vi "Annotate April.vi"(6 "hilight":bool, 7 "Annotate":bool, 9 "cutoffs":T1, 10 "Detected Tags":T3(array[cluster]), 11 "Refnum in":T2) -> (1 "margins":dbl[](array[numeric]), 2 "tags":T3(array[cluster]), 3 "Refnum out":T2)   [LabVIEW 2025]
uses:
  <vilib>/vision/Image Controls.llb/IMAQ Image.ctl
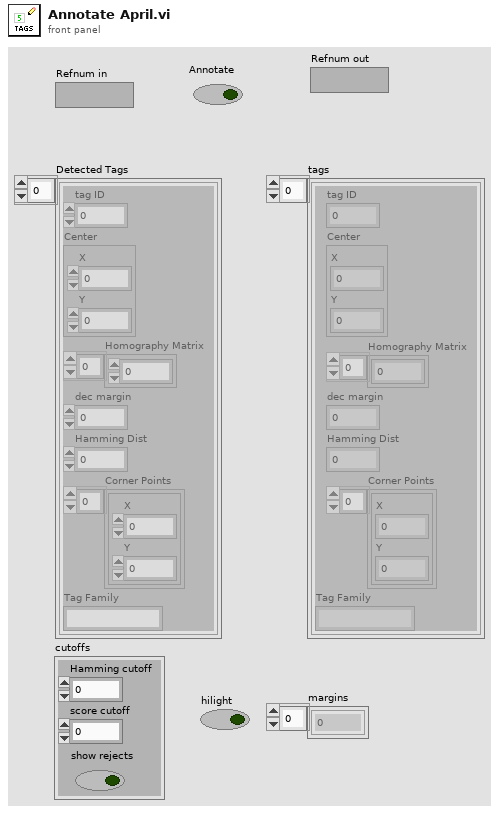
[diagram p1: front panel]
types:
  T1 = cluster{"Hamming cutoff":i32, "score cutoff":dbl, "show rejects":bool}
  T2 = typedef "IMAQ Image.ctl" = refnum<image>
  T3 = cluster{"tag ID":i32, "Center":cluster{"X":dbl, "Y":dbl}, "Homography Matrix":dbl[], "dec margin":dbl, "Hamming Dist":i32, "Corner Points":cluster{"X":dbl, "Y":dbl}[], "Tag Family":string}[]
  T4 = cluster{"Desired Font (Application)":enum16{"User-specified Font", "Application Font", "System Font", "Dialog Font"}, "[User-specified Font]":cluster{"Font Name":string, "Size":i16, "Strikeout?":bool, "Italic?":bool, "Underline?":bool, "Outline?":bool, "Shadow?":bool, "Bold?":bool, "Rotation Angle":dbl}, "Horizontal Alignment":i16, "Vertical Alignment":i16}
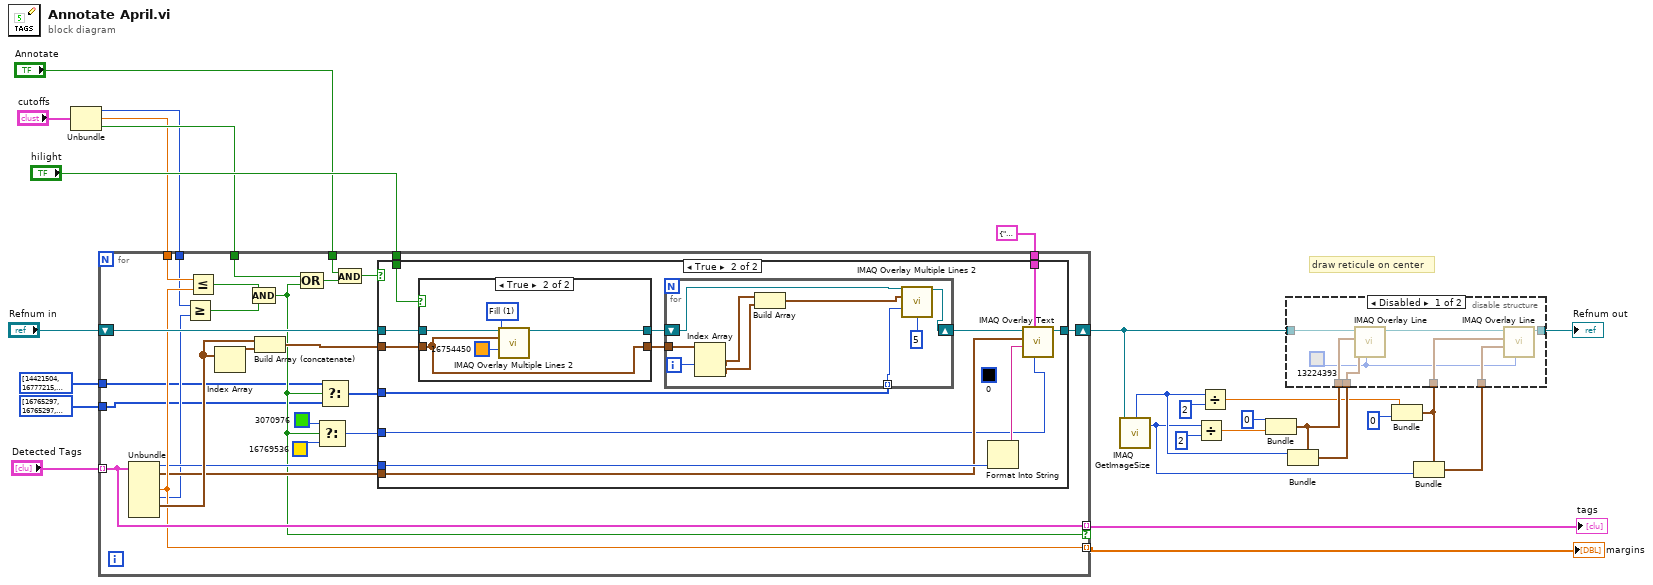
[diagram p0: block diagram]
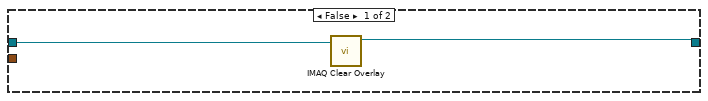
[diagram p3: hidden frame]
diagram:
  # "draw reticule on center"
  n1 = Unbundle("cutoffs") -> ("Hamming cutoff"=w4:i32, "score cutoff"=w5:dbl, "show rejects"=w6:bool)
  n2 = for {
    tunnel: "Detected Tags" -> [w51] mode=indexing
    shift-right: [w53] -> w22
    shift-left: "Refnum in" -> [w54]
    tunnel: [w51] -> w27 mode=indexing if=w32
    tunnel: [w50] -> w25 mode=indexing
    tunnel: w6 -> [w42]
    tunnel: T4 {"Desired Font (Application)"=enum."Application Font", "[User-specified Font]"={"Font Name"="", "Size"=12, "Strikeout?"=FALSE, "Italic?"=FALSE, "Underline?"=FALSE, "Outline?"=FALSE, "Shadow?"=FALSE, "Bold?"=FALSE, "Rotation Angle"=0.0}, "Horizontal Alignment"=1, "Vertical Alignment"=2} ("Font, Size & Style") -> [w39]
    tunnel: "hilight" -> [w38]
    tunnel: w5 -> [w37]
    tunnel: w4 -> [w35]
    tunnel: u32[] [14421504, 16777215, 16777215, 3070976] -> [w31]
    tunnel: u32[] [16765297, 16765297, 16765297, 16765297] -> [w30]
    tunnel: "Annotate" -> [w28]
    n3 = Unbundle(w51) -> ("tag ID"=w49:i32, "Center"=w48:cluster{"X":dbl, "Y":dbl}, "dec margin"=w50:dbl, "Hamming Dist"=w36:i32, "Corner Points"=w52:cluster{"X":dbl, "Y":dbl}[])  [unwired: 2 out]
    n4 = Greater Or Equal?(x=w35, y=w36) -> (x >= y?=w33:bool)
    n5 = Less Or Equal?(x=w37, y=w50) -> (x <= y?=w34:bool)
    n6 = Index Array(array=w52) -> (element=w44:cluster{"X":dbl, "Y":dbl})  [unwired: 1 in]
    n7 = Compound Arithmetic op=AND(w34, w33) -> (w32:bool)
    n8 = Build Array (concatenate)(w52, w44) -> (w43:cluster{"X":dbl, "Y":dbl}[])
    n9 = Compound Arithmetic op=OR(w42, w32) -> (w41:bool)
    n10 = Select(t=u32 3070976 ("Color"), s=w32, f=u32 16769536 ("Color")) -> (s? t:f=w45:u32)
    n11 = Select(t=w31, s=w32, f=w30) -> (s? t:f=w40:u32[])
    n12 = And(x=w28, y=w41) -> (x .and. y?=w29:bool)
    n13 = case shown="True" w29 {
      tunnel: w54 -> [w56 w60]
      tunnel: [w55 w69] -> w53
      tunnel: w49 -> [_ w68]
      tunnel: w48 -> [_ w67]
      tunnel: w45 -> [_ w63]
      tunnel: w43 -> [_ w61]
      tunnel: w40 -> [_ w65]
      tunnel: w39 -> [_ w64]
      tunnel: w38 -> [_ w57]
      frame False {
        n14 = call "IMAQ Clear Overlay"("Image"=w56) -> ("Image Out"=w55:T2)  [unwired: 9 in, 1 out]
      }
      frame True {
        (unwired) u32 0 ("Color")
        n15 = case shown="True" w57 {
          tunnel: w61 -> [w70 w73]
          tunnel: w60 -> [w71 w75]
          tunnel: [w71 w76] -> w59
          tunnel: [w70 w73] -> w58
          frame False {
          }
          frame True {
            w72 = u32 1 items=["Frame", "Fill"] ("Drawing Mode (Frame)")
            n16 = call "IMAQ Overlay Multiple Lines 2"("Image"=w75, "Line End Points"=w73, "Drawing Mode (Frame)"=w72, "Color"=u32 16754450) -> ("Image Out"=w76:T2)  [unwired: 10 in, 1 out]
          }
        }
        n17 = for {
          shift-right: [w81] -> w62
          shift-left: w59 -> [w80]
          tunnel: w58 -> [w85]
          tunnel: w65 -> [w77] mode=indexing
          i -> [w84]
          n18 = Index Array(array=w85, index #1=w84) -> (element #1=w82:cluster{"X":dbl, "Y":dbl}, element #2=w79:cluster{"X":dbl, "Y":dbl})  [unwired: 1 in]
          n19 = Build Array(w82, w79) -> (w83:cluster{"X":dbl, "Y":dbl}[])
          n20 = call "IMAQ Overlay Multiple Lines 2"("Image"=w80, "Line End Points"=w83, "Color"=w77, "Width"=u32 5) -> ("Image Out"=w81:T2)  [unwired: 10 in, 1 out]
        }
        n21 = Format Into String(w68) -> (resulting string=w66:string)  [unwired: 3 in, 1 out]
        n22 = call "IMAQ Overlay Text"("Text Color (black)"=w63, "Font, Size & Style"=w64, "String"=w66, "Origin"=w67, "Image"=w62) -> ("Image Out"=w69:T2)  [unwired: 5 in, 1 out]
      }
    }
  }
  "tags" <- w27
  "margins" <- w25
  n23 = call "IMAQ GetImageSize"("Image"=w22) -> ("Y Resolution"=w12:i32, "X Resolution"=w17:i32)  [unwired: 3 in, 1 out]
  n24 = Divide(x=w12, y=2 ("X")) -> (x/y=w19:dbl)
  n25 = Divide(x=w17, y=2 ("X")) -> (x/y=w13:dbl)
  n26 = Bundle("X"=0, w19) -> (w18:cluster{"X":i32, dbl})  [unwired: 1 in]
  n27 = Bundle(cluster=w18, "X"=w17) -> (w16:cluster{"X":i32, dbl})  [unwired: 1 in]
  n28 = Bundle(w13, "X"=0) -> (w10:cluster{dbl, "X":i32})  [unwired: 1 in]
  n29 = Bundle(cluster=w10, "X"=w12) -> (w11:cluster{dbl, "X":i32})  [unwired: 1 in]
  n30 = disable-structure shown="Disabled" {
    disable-tunnel: [w92 w94] -> w23
    disable-tunnel: w22 -> [w91 w94]
    disable-tunnel: w18 -> [w90 _]
    disable-tunnel: w16 -> [w89 _]
    disable-tunnel: w11 -> [w88 _]
    disable-tunnel: w10 -> [w87 _]
    frame Disabled {
      w86 = u32 13224393 ("Color")
      n31 = call "IMAQ Overlay Line"("Color"=w86, "End Point"=w89, "Start Point"=w90, "Image"=w91) -> ("Image Out"=w93:T2)  [unwired: 6 in, 1 out]
      n32 = call "IMAQ Overlay Line"("Color"=w86, "End Point"=w88, "Start Point"=w87, "Image"=w93) -> ("Image Out"=w92:T2)  [unwired: 6 in, 1 out]
    }
    frame Enabled {
    }
  }
  "Refnum out" <- w23
